vi "BasicLogger.vi"(4 "indicator":refnum<vi>, 5 "error in":errorcluster, 8 "text":string) -> (0 "error out":errorcluster, 3 "recent":string[](array[string]))   [LabVIEW 2010]
panel:
  in  "log_length":i32=20
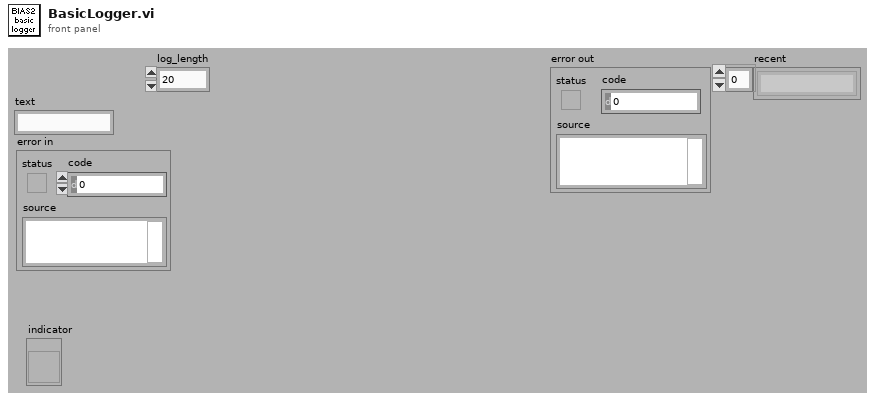
[diagram p1: front panel]
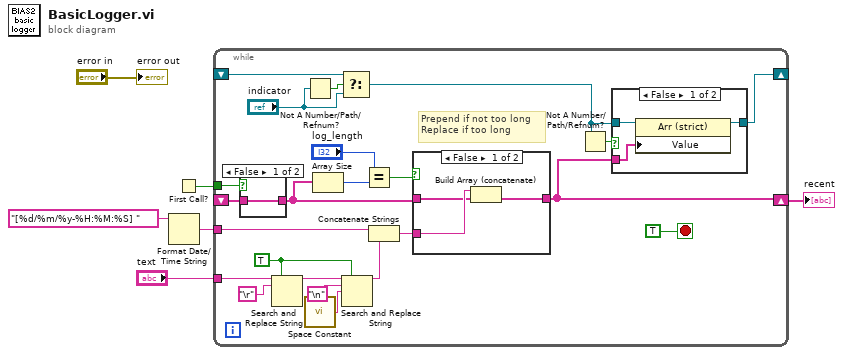
[diagram p0: block diagram]
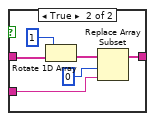
[diagram p2: hidden frame]
diagram:
  n1 = Format Date/Time String(time format string (%c)="[%d/%m/%y-%H:%M:%S] ") -> (date/time string=w2:string)  [unwired: 2 in]
  n2 = First Call?() -> (First Call?: T/F=w4:bool)
  n3 = while {
    tunnel: w4 -> [w29]
    shift-right: [w26] -> w6
    shift-left: _ -> [w24]
    shift-right: [w27] -> _
    shift-left: _ -> [w20]
    tunnel: w2 -> [w18]
    tunnel: "text" -> [w17]
    stop <- TRUE stop-if-true
    w9 = TRUE ("replace all? (F)")
    # "Prepend if not too long\nReplace if too long"
    n4 = case shown="False" w29 {
      tunnel: w24 -> [w43 _]
      tunnel: [w43 _] -> w23
      frame False {
      }
      frame True {
      }
    }
    n5 = Search and Replace String(replace all?=w9, input string=w17, search string="\r") -> (result string=w11:string)  [unwired: 5 in, 3 out]
    n6 = Not A Number/Path/Refnum?(number/path/refnum="indicator") -> (NaN/Path/Refnum?=w22:bool)
    n7 = call <vilib>:"Space Constant.vi"() -> ("String"=w13:string)
    n8 = Array Size(array=w23) -> (size(s)=w16:i32)
    n9 = Select(t=w20, s=w22, f="indicator") -> (s? t:f=w21:refnum<vi>)
    n10 = Search and Replace String(replace all?=w9, input string=w11, search string="\n", replace string=w13) -> (result string=w7:string)  [unwired: 4 in, 3 out]
    n11 = Equal?(x="log_length", y=w16) -> (x = y?=w14:bool)
    n12 = Concatenate Strings(w18, w7) -> (w8:string)
    n13 = case shown="False" w14 {
      tunnel: w23 -> [w30 w38]
      tunnel: w8 -> [w31 w34]
      tunnel: [w32 w35] -> w26
      frame False {
        n14 = Build Array (concatenate)(w31, w30) -> (w32:string[])
      }
      frame True {
        n15 = Rotate 1D Array(1:w38, 2:1 ("n")) -> (0:w36:string[])
        n16 = Replace Array Subset(array=w36, new element=w34, index=0) -> (w35:string[])
      }
    }
    n17 = Not A Number/Path/Refnum?(number/path/refnum=w21) -> (NaN/Path/Refnum?=w25:bool)
    n18 = case shown="False" w25 {
      tunnel: [w41 w42] -> w27
      tunnel: w26 -> [w40 _]
      tunnel: w21 -> [w39 w42]
      frame False {
        n19 = property class="Arr (strict)"(reference=w39, "Value"=w40) -> (reference out=w41:refnum<vi>)  [unwired: 1 in, 1 out]
      }
      frame True {
      }
    }
  }
  "recent" <- w6
  "error out" <- "error in"
